vi "CRYGet Data Infomation.vi"(9 "Graph Type":string="XY", 11 "Data Names":string[](array[string])) -> (0 "Result Rows":i32[](array[numeric]), 1 "Color Array":u32[](array[colorbox]), 2 "Value Rows":i32[](array[numeric]), 3 "Rows":i32[](array[numeric]))   [LabVIEW 2013]
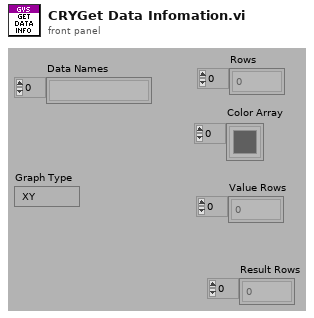
[diagram p1: front panel]
types:
  T1 = typedef "CRYData Cluster.ctl" = cluster{"Name":string, "Curve":cluster{"x":dbl, "y":dbl, "z":dbl}[], "X data":u16, "Y data":u16, "Z data":u16, "X axis":u16, "Y axis":u16, "Z axis":u16, "X unit":string, "Y unit":string, "Z unit":string, "X dB ref":dbl, "Y dB ref":dbl, "Z dB ref":dbl, "single val":bool, "protected":bool, "display X":bool, "display Y":bool, "display Z":bool, "Test Info":string, "Step No.":i32, "Plot Settings":cluster{"Color":u32, "Interpolation":u8, "Point Style":u8, "Line Style":u8, "Point Color":u32, "Line Width":u8, "Bar Plot Style":u8, "Fill To":i16}, "AutoProtect":bool}
  T2 = typedef "CRYWaveform Cluster.ctl" = cluster{"Waveform":cluster{"X0":dbl, "dX":dbl, "Y":sgl[]}, "X data":u16, "Y data":u16, "Y axis":u16, "X unit":string, "Y unit":string, "Y dB ref":dbl, "display Y":bool, "display X":bool, "Overload?":bool, "Test Info":string, "Step No.":i32, "Name":string, "protected":bool, "Sqc history":string[], "Signal Channel ID":i32, "Plot Settings":cluster{"Color":u32, "Interpolation":u8, "Point Style":u8, "Line Style":u8, "Point Color":u32, "Line Width":u8, "Bar Plot Style":u8, "Fill To":i16}, "AutoProtect":bool}
  T3 = typedef "CRYResult Cluster.ctl" = cluster{"Name":string, "Margin":dbl, "unit":string, "Verdict":bool, "Limit":string, "Max/Min":string, "protected":bool, "Step No.":i32, "Test Info":string, "AutoProtect":bool}
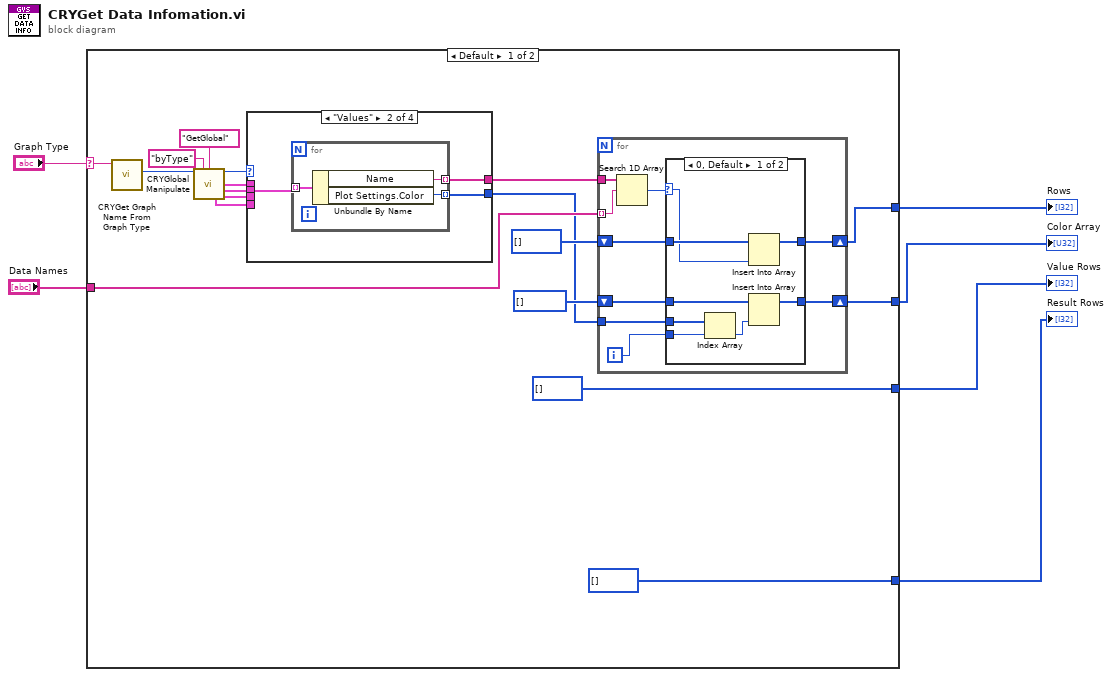
[diagram p0: block diagram]
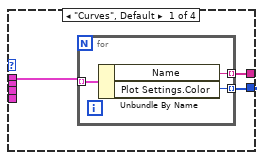
[diagram p3: hidden frame]
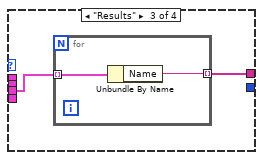
[diagram p4: hidden frame]
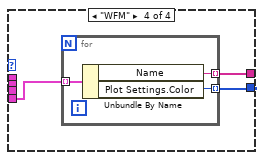
[diagram p5: hidden frame]
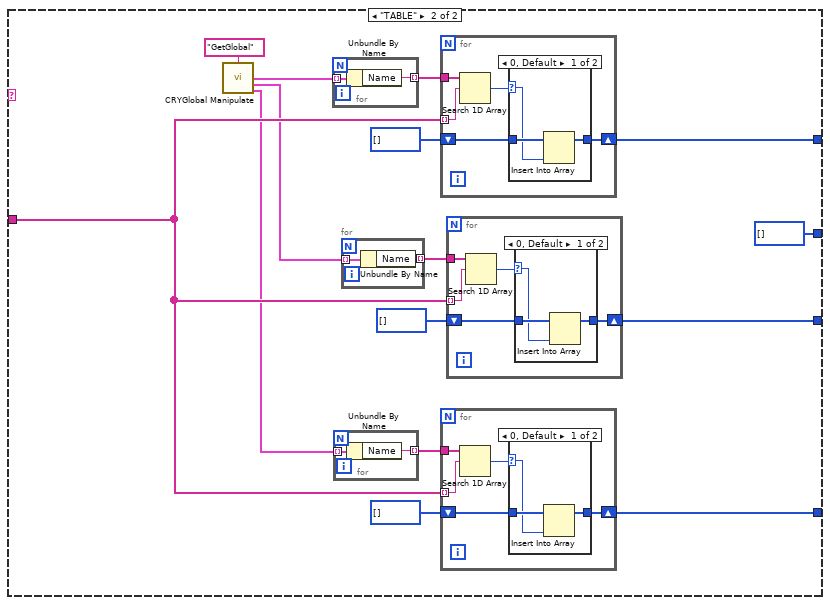
[diagram p6: hidden frame]
diagram:
  n1 = case shown="Default" "Graph Type" {
    selector: "Graph Type" -> [w23 _]
    tunnel: "Data Names" -> [w18 w72]
    tunnel: [w16 w78] -> w3
    tunnel: [i32[] [] ("Rows") w75] -> w5
    tunnel: [i32[] [] ("Rows") w71] -> w1
    tunnel: [w15 u32[] [] ("Color Array")] -> w2
    frame Default {
      n2 = call "CRYGet Graph Name From Graph Type.vi"("Graph Type"=w23) -> ("Type"=w13:enum16{"Curves", "Values", "Results", "WFM"})  [unwired: 10 out]
      n3 = call "CRYGlobal Manipulate.vi"("Type"=w13, "sOption"="byType", "sAction"="GetGlobal") -> ("Type out"=w12:enum16{"Curves", "Values", "Results", "WFM"}, "Curves Out"=w11:T1[], "Values Out"=w10:T1[], "WFM Out"=w8:T2[], "Results Out"=w9:T3[])  [unwired: 6 in, 2 out]
      n4 = case shown="\"Values\"" w12 {
        tunnel: [w46 w52 w57 w62] -> w19
        tunnel: [w45 w51 _ w61] -> w17
        tunnel: w11 -> [w44 _ _ _]
        tunnel: w10 -> [_ w50 _ _]
        tunnel: w9 -> [_ _ w56 _]
        tunnel: w8 -> [_ _ _ w60]
        frame "Curves", Default {
          n5 = for {
            tunnel: w44 -> [w49] mode=indexing
            tunnel: [w48] -> w46 mode=indexing
            tunnel: [w47] -> w45 mode=indexing
            n6 = Unbundle By Name(w49) -> ("Name"=w48:string, "Plot Settings.Color"=w47:u32)
          }
        }
        frame "Values" {
          n7 = for {
            tunnel: w50 -> [w55] mode=indexing
            tunnel: [w54] -> w52 mode=indexing
            tunnel: [w53] -> w51 mode=indexing
            n8 = Unbundle By Name(w55) -> ("Name"=w54:string, "Plot Settings.Color"=w53:u32)
          }
        }
        frame "Results" {
          n9 = for {
            tunnel: w56 -> [w59] mode=indexing
            tunnel: [w58] -> w57 mode=indexing
            n10 = Unbundle By Name(w59) -> ("Name"=w58:string)
          }
        }
        frame "WFM" {
          n11 = for {
            tunnel: w60 -> [w65] mode=indexing
            tunnel: [w64] -> w62 mode=indexing
            tunnel: [w63] -> w61 mode=indexing
            n12 = Unbundle By Name(w65) -> ("Name"=w64:string, "Plot Settings.Color"=w63:u32)
          }
        }
      }
      n13 = for {
        tunnel: w18 -> [w33] mode=indexing
        tunnel: w19 -> [w32]
        shift-right: [w29] -> w15
        shift-left: u32[] [] ("Color Array") -> [w30]
        tunnel: w17 -> [w28]
        shift-right: [w26] -> w16
        shift-left: i32[] [] ("Rows") -> [w27]
        i -> [w25]
        n14 = Search 1D Array(1D array=w32, element=w33) -> (index of element=w31:i32)  [unwired: 1 out]
        n15 = case shown="0, Default" w31 {
          selector: w31 -> [w34 _]
          tunnel: [w40 w43] -> w29
          tunnel: w30 -> [w41 w43]
          tunnel: w28 -> [w36 _]
          tunnel: w27 -> [w39 w42]
          tunnel: [w38 w42] -> w26
          tunnel: w25 -> [w37 _]
          frame 0, Default {
            n16 = Index Array(array=w36, index=w37) -> (element=w35:u32)
            n17 = Insert Into Array(array=w39, new element=w34) -> (w38:i32[])  [unwired: 1 in]
            n18 = Insert Into Array(array=w41, new element=w35) -> (w40:u32[])  [unwired: 1 in]
          }
          frame -1 {
          }
        }
      }
    }
    frame "TABLE" {
      n19 = call "CRYGlobal Manipulate.vi"("sAction"="GetGlobal") -> ("Curves Out"=w68:T1[], "Values Out"=w67:T1[], "Results Out"=w66:T3[])  [unwired: 8 in, 4 out]
      n20 = for {
        tunnel: w68 -> [w113] mode=indexing
        tunnel: [w112] -> w79 mode=indexing
        n21 = Unbundle By Name(w113) -> ("Name"=w112:string)
      }
      n22 = for {
        tunnel: w66 -> [w102] mode=indexing
        tunnel: [w101] -> w77 mode=indexing
        n23 = Unbundle By Name(w102) -> ("Name"=w101:string)
      }
      n24 = for {
        tunnel: w67 -> [w91] mode=indexing
        tunnel: [w90] -> w74 mode=indexing
        n25 = Unbundle By Name(w91) -> ("Name"=w90:string)
      }
      n26 = for {
        tunnel: w72 -> [w107] mode=indexing
        tunnel: w79 -> [w106]
        shift-right: [w103] -> w78
        shift-left: i32[] [] ("Rows") -> [w104]
        n27 = Search 1D Array(1D array=w106, element=w107) -> (index of element=w105:i32)  [unwired: 1 out]
        n28 = case shown="0, Default" w105 {
          selector: w105 -> [w108 _]
          tunnel: w104 -> [w110 w111]
          tunnel: [w109 w111] -> w103
          frame 0, Default {
            n29 = Insert Into Array(array=w110, new element=w108) -> (w109:i32[])  [unwired: 1 in]
          }
          frame -1 {
          }
        }
      }
      n30 = for {
        tunnel: w72 -> [w96] mode=indexing
        tunnel: w77 -> [w95]
        shift-right: [w92] -> w75
        shift-left: i32[] [] ("Rows") -> [w93]
        n31 = Search 1D Array(1D array=w95, element=w96) -> (index of element=w94:i32)  [unwired: 1 out]
        n32 = case shown="0, Default" w94 {
          selector: w94 -> [w97 _]
          tunnel: w93 -> [w99 w100]
          tunnel: [w98 w100] -> w92
          frame 0, Default {
            n33 = Insert Into Array(array=w99, new element=w97) -> (w98:i32[])  [unwired: 1 in]
          }
          frame -1 {
          }
        }
      }
      n34 = for {
        tunnel: w72 -> [w85] mode=indexing
        tunnel: w74 -> [w84]
        shift-right: [w81] -> w71
        shift-left: i32[] [] ("Rows") -> [w82]
        n35 = Search 1D Array(1D array=w84, element=w85) -> (index of element=w83:i32)  [unwired: 1 out]
        n36 = case shown="0, Default" w83 {
          selector: w83 -> [w86 _]
          tunnel: w82 -> [w88 w89]
          tunnel: [w87 w89] -> w81
          frame 0, Default {
            n37 = Insert Into Array(array=w88, new element=w86) -> (w87:i32[])  [unwired: 1 in]
          }
          frame -1 {
          }
        }
      }
    }
  }
  "Color Array" <- w2
  "Rows" <- w3
  "Value Rows" <- w1
  "Result Rows" <- w5
